vi "get_key_value_from_string.vi"(0 "key groups":string[](array[string])=["SET_PID", "SET_OUTPUT"], 1 "input string":string) -> (2 "key list":string[](array[string]), 3 "key index list":i32[](array[numeric]), 4 "value list":string[](array[string]))   [LabVIEW 2016]
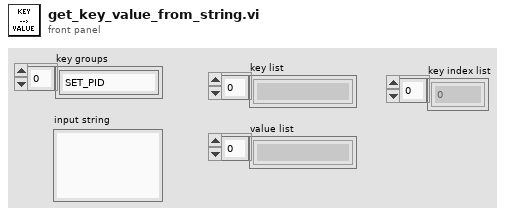
[diagram p1: front panel]
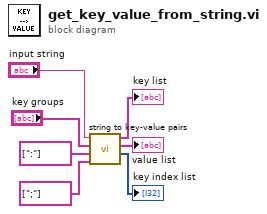
[diagram p0: block diagram]
diagram:
  n1 = call "string to key-value pairs.vi"("separator between key-value pairs"=string[] [";"], "separator between key and value"=string[] [":"], "known key list"="key groups", "input string"="input string") -> ("key index list"=→"key index list":i32[], "value list"=→"value list":string[], "key list"=→"key list":string[])  [unwired: 1 in]
